vi "FGEN DC voltage.vi"(9 "Output voltage (V)":dbl, 11 "Resource Name":refnum<k15>="PXI1Slot2") -> (0 "error out":errorcluster)   [LabVIEW 2018]
uses:
  <instrlib>/niFgen/niFgen.llb/niFgen Output Mode.ctl
  <instrlib>/niFgen/niFgen.llb/niFgen Create Waveform (I16).vi
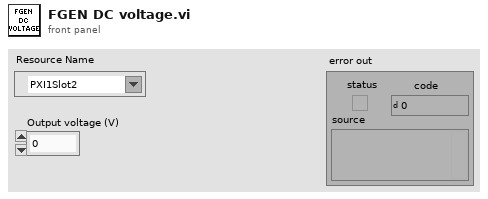
[diagram p1: front panel]
types:
  T1 = typedef "niFgen Output Mode.ctl" = u32
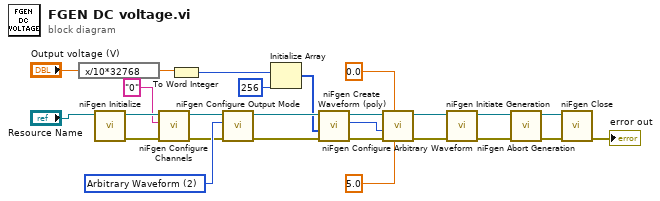
[diagram p0: block diagram]
diagram:
  w26 = T1 2 items=["Standard Function", "Frequency List", "Arbitrary Waveform", "Arbitrary Sequence", "Script"] ("Output Mode (default: 0=Standard Function)")
  n1 = expression code="x/10*32768"("Output voltage (V)") -> (w10:dbl)
  n2 = call <instrlib>:"niFgen Initialize.vi"("Resource Name"="Resource Name") -> ("error out"=w6:errorcluster, "Instrument Handle Out"=w5:refnum<k15>)  [unwired: 9 in]
  n3 = call <instrlib>:"niFgen Configure Channels.vi"("error in (no error)"=w6, "Channels"="0" ("Channel Name"), "Instrument Handle"=w5) -> ("error out"=w1:errorcluster, "Instrument Handle Out"=w2:refnum<k15>)  [unwired: 7 in]
  n4 = To Word Integer(number=w10) -> (16bit integer=w9:i16)
  n5 = call <instrlib>:"niFgen Configure Output Mode.vi"("error in (no error)"=w1, "Output Mode (default: 0=Standard Function)"=w26, "Instrument Handle"=w2) -> ("error out"=w19:errorcluster, "Instrument Handle Out"=w20:refnum<k15>)  [unwired: 6 in]
  n6 = Initialize Array(w9, 256 ("dimension size")) -> (w12:i16[])
  n7 = call-poly <instrlib>:"niFgen Create Waveform (poly).vi"("error in (no error)"=w19, "Waveform Data Array"=w12, "Instrument Handle"=w20) -> ("error out"=w18:errorcluster, "Waveform Handle"=w14:i32, "Instrument Handle Out"=w17:refnum<k15>)  [unwired: 6 in]
  n8 = call <instrlib>:"niFgen Configure Arbitrary Waveform.vi"("Gain"=5.0, "Offset"=0.0, "error in (no error)"=w18, "Waveform Handle"=w14, "Instrument Handle"=w17) -> ("error out"=w15:errorcluster, "Instrument Handle Out"=w16:refnum<k15>)  [unwired: 5 in]
  n9 = call <instrlib>:"niFgen Initiate Generation.vi"("error in (no error)"=w15, "Instrument Handle"=w16) -> ("error out"=w22:errorcluster, "Instrument Handle Out"=w23:refnum<k15>)  [unwired: 8 in]
  n10 = call <instrlib>:"niFgen Abort Generation.vi"("error in (no error)"=w22, "Instrument Handle"=w23) -> ("error out"=w24:errorcluster, "Instrument Handle Out"=w25:refnum<k15>)  [unwired: 8 in]
  n11 = call <instrlib>:"niFgen Close.vi"("error in (no error)"=w24, "Instrument Handle"=w25) -> ("error out"=→"error out":errorcluster)  [unwired: 9 in]
